vi "GraphSetting Plot (Wave).vi"(6 "コマンド":T1, 8 "error in (no error)":errorcluster caption="err(in)", 9 "アクティブプロット":u16, 10 "プロット(in)":T2 {"Yスケール" items=["振幅1234", "振幅 2", "振幅 33"]; "Xスケール" items=["XX"]; "プロット補間" max=5 step=1; "ポイントスタイル" max=16 step=1; "太さ" max=5 step=1; "ラインスタイル" max=4 step=1}, 11 "波形グラフref(in)":refnum<vi>) -> (0 "error out":errorcluster caption="err(out)", 2 "プロット(out)":T2 {"Yスケール" items=["振幅1234", "振幅 2", "振幅 33"]; "Xスケール" items=["XX"]; "プロット補間" max=5 step=1; "ポイントスタイル" max=16 step=1; "太さ" max=5 step=1; "ラインスタイル" max=4 step=1})   [LabVIEW 2016]
uses:
  TypeDef/GraphSetting Plot.ctl
  TypeDef/GraphSetting Command.ctl
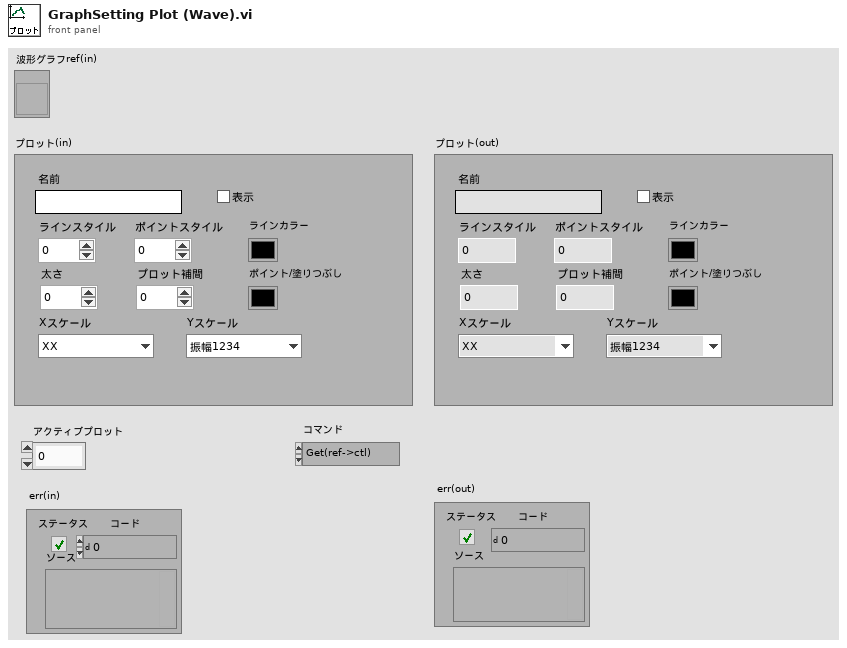
[diagram p1: front panel]
types:
  T1 = typedef "GraphSetting Command.ctl" = enum16{"Get(ref->ctl)", "Set(ctl->ref)"}
  T2 = typedef "GraphSetting Plot.ctl" = cluster{"名前":string, "表示":bool, "ラインスタイル":u8, "太さ":u8, "ポイントスタイル":u8, "プロット補間":u8, "ラインカラー":u32, "ポイント/塗りつぶし":u32, "Xスケール":u16, "Yスケール":u16}
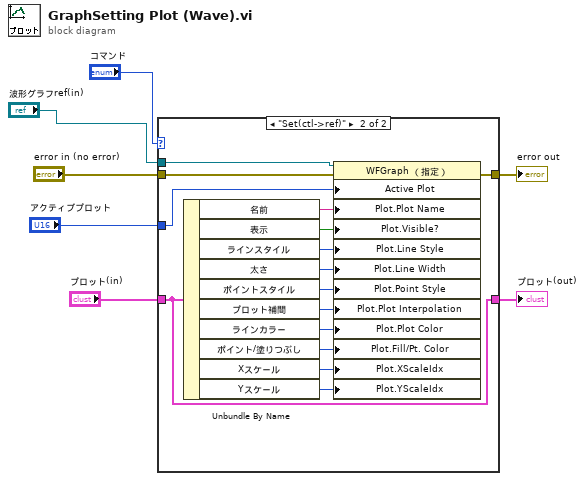
[diagram p0: block diagram]
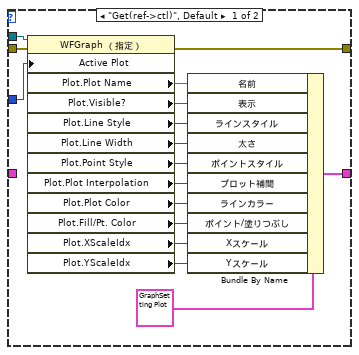
[diagram p2: hidden frame]
diagram:
  n1 = case shown="\"Set(ctl->ref)\"" "コマンド" {
    tunnel: "アクティブプロット" -> [w12 w38]
    tunnel: "波形グラフref(in)" -> [w11 w24]
    tunnel: [w10 w25] -> w6
    tunnel: "プロット(in)" -> [_ w25]
    tunnel: [w8 w27] -> w3
    tunnel: "error in (no error)" -> [w9 w26]
    frame "Get(ref->ctl)", Default {
      n2 = property class="WFGraph （指定）"(reference=w11, error in=w9, "Active Plot"=w12) -> (error out=w8:errorcluster, "Plot.Plot Name"=w13:string, "Plot.Visible?"=w14:bool, "Plot.Line Style"=w15:u8, "Plot.Line Width"=w16:u8, "Plot.Point Style"=w17:u8, "Plot.Plot Interpolation"=w18:u8, "Plot.Plot Color"=w19:u32, "Plot.Fill/Pt. Color"=w20:u32, "Plot.XScaleIdx"=w21:u32, "Plot.YScaleIdx"=w22:u32)  [unwired: 1 out]
      n3 = Bundle By Name(cluster=T2 {"名前"="プロット0aa", "表示"=TRUE, "ラインスタイル"=0, "太さ"=0, "ポイントスタイル"=0, "プロット補間"=2, "ラインカラー"=14467840, "ポイント/塗りつぶし"=16448250, "Xスケール"=0, "Yスケール"=0} ("プロット"), "名前"=w13, "表示"=w14, "ラインスタイル"=w15, "太さ"=w16, "ポイントスタイル"=w17, "プロット補間"=w18, "ラインカラー"=w19, "ポイント/塗りつぶし"=w20, "Xスケール"=w21, "Yスケール"=w22) -> (w10:T2)
    }
    frame "Set(ctl->ref)" {
      n4 = Unbundle By Name(w25) -> ("名前"=w37:string, "表示"=w36:bool, "ラインスタイル"=w35:u8, "太さ"=w34:u8, "ポイントスタイル"=w33:u8, "プロット補間"=w32:u8, "ラインカラー"=w31:u32, "ポイント/塗りつぶし"=w30:u32, "Xスケール"=w29:u16, "Yスケール"=w28:u16)
      n5 = property class="WFGraph （指定）"(reference=w24, error in=w26, "Active Plot"=w38, "Plot.Plot Name"=w37, "Plot.Visible?"=w36, "Plot.Line Style"=w35, "Plot.Line Width"=w34, "Plot.Point Style"=w33, "Plot.Plot Interpolation"=w32, "Plot.Plot Color"=w31, "Plot.Fill/Pt. Color"=w30, "Plot.XScaleIdx"=w29, "Plot.YScaleIdx"=w28) -> (error out=w27:errorcluster)  [unwired: 1 out]
    }
  }
  "プロット(out)" <- w6
  "error out" <- w3
